vi "PathPlanner_GeomUtil_TranslationLerp.vi"(9 "T":dbl, 10 "EndVal":T1 {"Y" format="%14.3f"; "X" format="%14.3f"}, 11 "StartVal":T1 {"Y" format="%14.3f"; "X" format="%14.3f"}) -> (3 "Lerp":T1 {"Y" format="%14.3f"; "X" format="%14.3f"})   [LabVIEW 2019, in "PathPlanner.lvlib"]
doc: "Inputs: \n - a - translation2d - Position 1\n - b - translation2d - Position 2\n - t - double - Interpolation factor (0.0-1.0)\n\nOutputs:\n - lerp - translation2d - Interpolated value"
uses:
  PathPlanner.lvlib
  <vilib>/Rock Robotics/WPI/ThirdParty/JAS_Junk/TrajLib/TypeDef/TRANSLATION2D.ctl
  <vilib>/Rock Robotics/WPI/ThirdParty/JAS_Junk/TrajLib/Translation2d_Create.vi
  <vilib>/Rock Robotics/WPI/ThirdParty/JAS_Junk/TrajLib/Trajectory_Library.lvlib
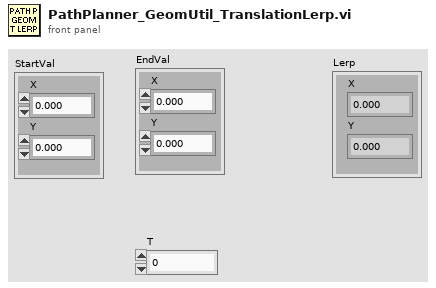
[diagram p1: front panel]
types:
  T1 = typedef "Trajectory_Library.lvlib/TRANSLATION2D.ctl" = cluster{"X":dbl, "Y":dbl}
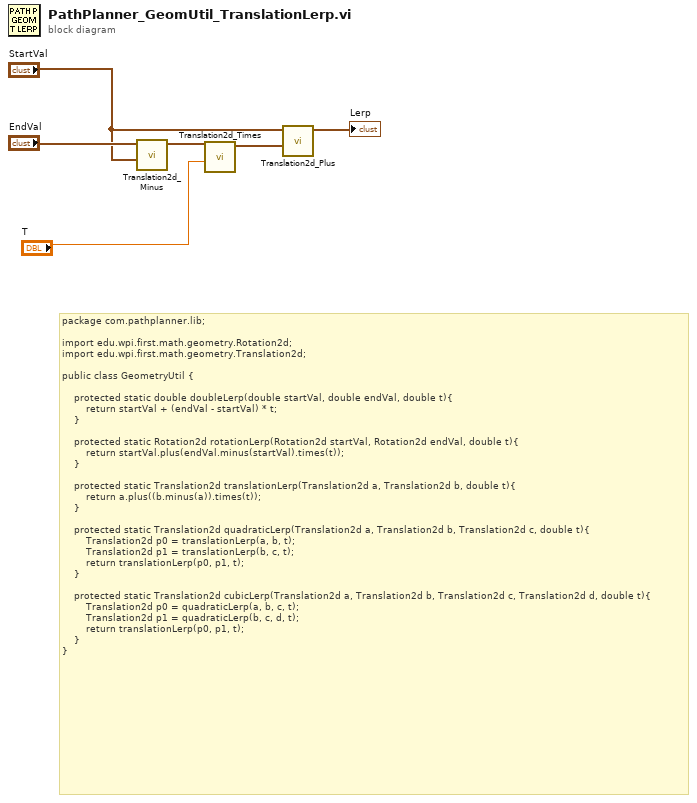
[diagram p0: block diagram]
diagram:
  # "package com.pathplanner.lib;\n\nimport edu.wpi.first.math.geometry.Rotation2d;\nimport edu.wpi.first.math.geometry.Translation2d;\n\npublic class GeometryUtil {\n\n    protected static double doubleLerp(double startVal, double endVal, double t){\n        return startVal + (endVal - startVal) * t;\n    }\n\n    protected static Rotation2d rotationLerp(Rotation2d startVal, Rotation2d endVal, double t){\n        return startVal.plus(endVal.minus(startVal).times(t));\n    }\n\n    protected static Translation2d translationLerp(Translation2d a, Translation2d b, double t){\n        return a.plus((b.minus(a)).times(t));\n    }\n\n    protected static Translation2d quadraticLerp(Translation2d a, Translation2d b, Translation2d c, double t){\n        Translation2d p0 = translationLerp(a, b, t);\n        Translation2d p1 = translationLerp(b, c, t);\n        return translationLerp(p0, p1, t);\n    }\n\n    protected static Translation2d cubicLerp(Translation2d a, Translation2d b, Translation2d c, Translation2d d, double t){\n        Translation2d p0 = quadraticLerp(a, b, c, t);\n        Translation2d p1 = quadraticLerp(b, c, d, t);\n        return translationLerp(p0, p1, t);\n    }\n}"
  n1 = call <vilib>:"Translation2d_Minus.vi"("other Translation"="StartVal", "In Translation"="EndVal") -> ("Out Translation"=w5:T1)  [unwired: 9 in]
  n2 = call <vilib>:"Translation2d_Times.vi"("Scalar"="T", "In Translation"=w5) -> ("Out Translation"=w2:T1)  [unwired: 9 in]
  n3 = call <vilib>:"Translation2d_Plus.vi"("other Translation"=w2, "In Translation"="StartVal") -> ("Out Translation"=→"Lerp":T1)  [unwired: 9 in]
